vi "PDC_GetExternalOutMode.vi"(8 "error in (no error)":errorcluster, 10 "Port":u32, 11 "DeviceNo":u32) -> (0 "error out":errorcluster, 2 "Mode":u32, 3 "ReturnValue":u32, 4 "ErrorCode":u32)   [LabVIEW 2015]
doc: "This VI retrieves the output signal settings of the specified device."
uses:
  PDCLIB.dll
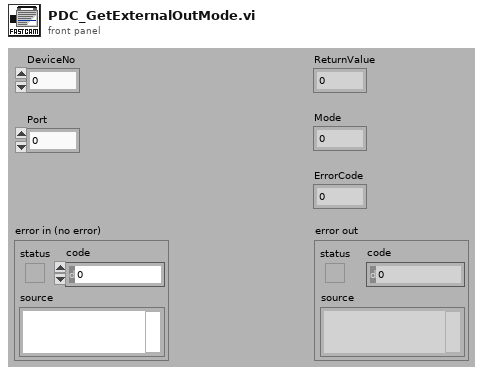
[diagram p1: front panel]
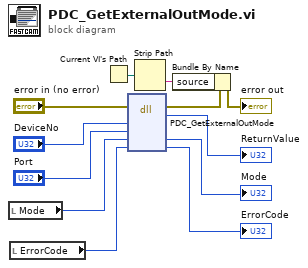
[diagram p0: block diagram]
diagram:
  n1 = local read "Mode"() -> (w6:u32)
  n2 = local read "ErrorCode"() -> (w9:u32)
  n3 = Current VI's Path() -> (path=w3:path)
  n4 = dll-call lib="PDCLIB.dll" fn="PDC_GetExternalOutMode"(error in="error in (no error)", "nDeviceNo"="DeviceNo", "nPort"="Port", "pMode"=w6, "pErrorCode"=w9) -> (error out=w2:errorcluster, "return type"=→"ReturnValue":u32, "pMode"=→"Mode":u32, "pErrorCode"=→"ErrorCode":u32)  [unwired: 4 in, 1 out]
  n5 = Strip Path(path=w3) -> (name=w4:string)  [unwired: 1 out]
  n6 = Bundle By Name(cluster=w2, "source"=w4) -> (→"error out":errorcluster)
